vi "Enqueue--complete_tour_found.vi"(8 "error in (no error)":errorcluster, 11 "completed_tour":T1) -> (0 "error out":errorcluster)   [LabVIEW 2020, in "main.lvlib"]
doc: "Blank VI with error handling."
uses:
  main.lvlib
  core/core_data/completed_tour.ctl
  core/core_data/chessboard_index.ctl
  core/core_data/tour type (enum).ctl
  core/core_data/core_data.lvlib
panel:
  # "Development\ncontrols/indicators useful for development and testing, but which are not outputs of the VI"
  # "Input\nInputs to the VI"
  # "Output\nOutputs of the VI"
  # "Description\n\nBlank VI with error handling case. \n\nSummarize the use of this VI in this space."
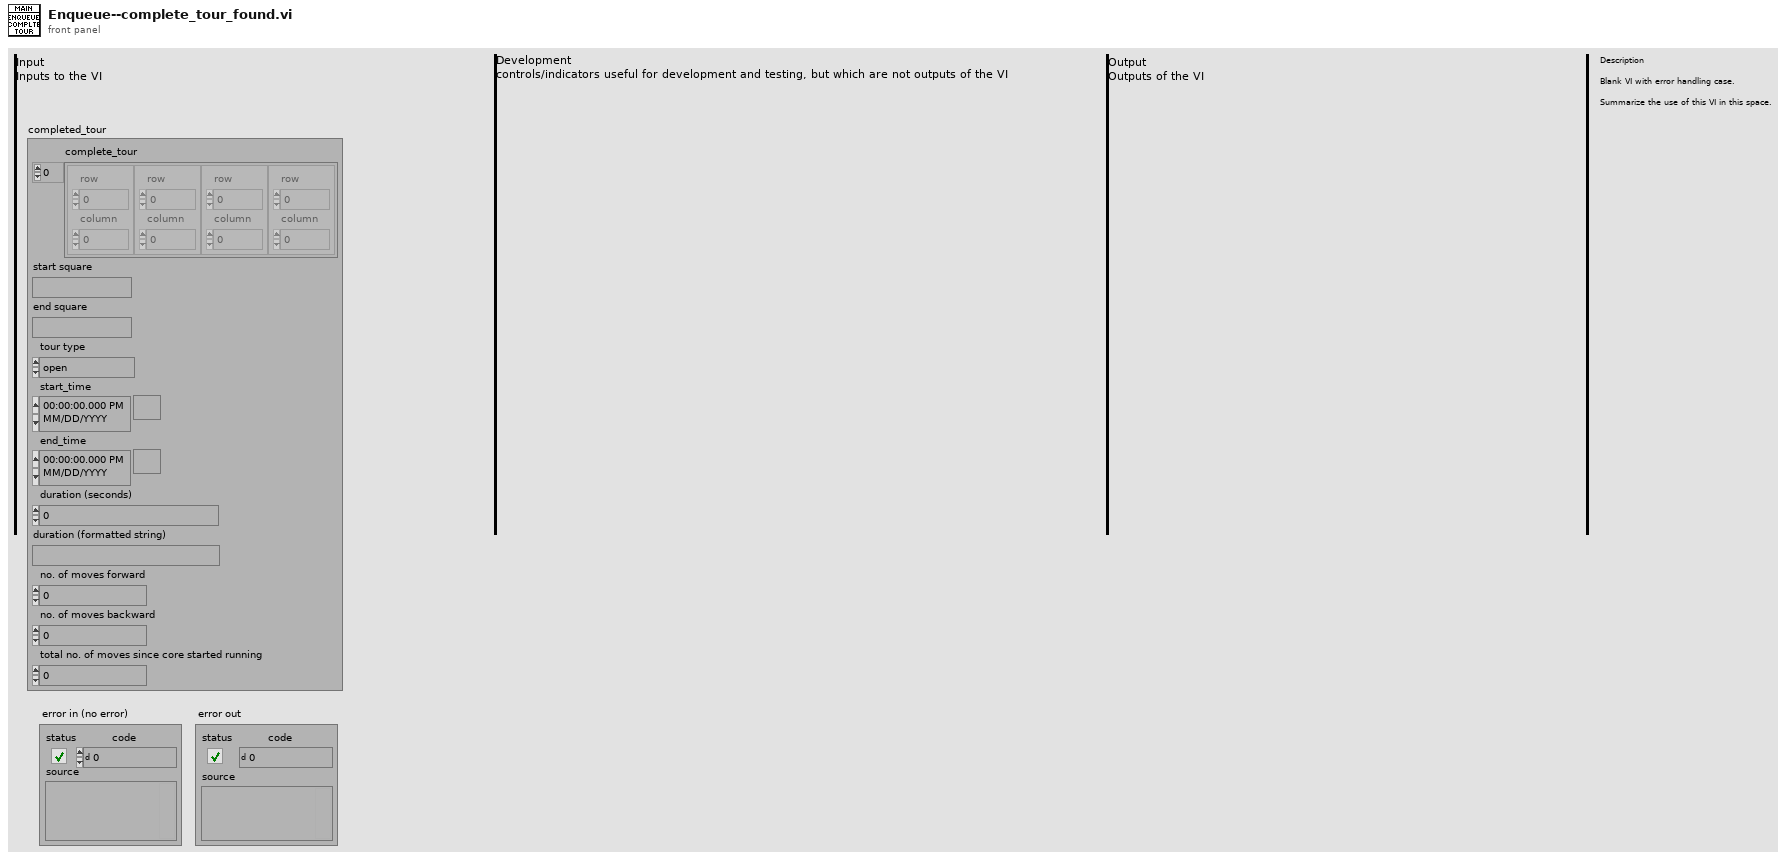
[diagram p1: front panel]
types:
  T1 = typedef "core.lvlib/core_data.lvlib/completed_tour.ctl" = cluster{"complete_tour":T2[], "start square":string, "end square":string, "tour type":T3, "start_time":timestamp, "end_time":timestamp, "duration (seconds)":dbl, "duration (formatted string)":string, "no. of moves forward":u64, "no. of moves backward":u64, "total no. of moves since core started running":u64}
  T2 = typedef "core.lvlib/core_data.lvlib/chessboard_index.ctl" = cluster{"row":u8, "column":u8}
  T3 = typedef "core.lvlib/core_data.lvlib/tour type (enum).ctl" = enum16{"open", "closed"}
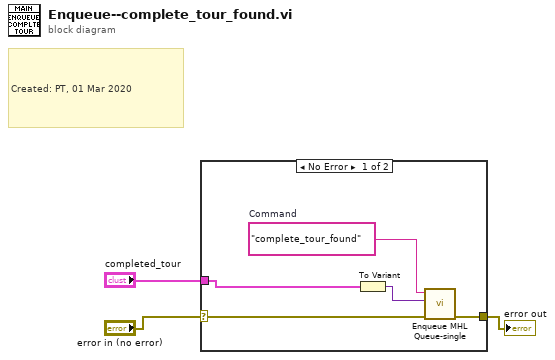
[diagram p0: block diagram]
diagram:
  # "Created: PT, 01 Mar 2020"
  n1 = case shown="No Error" "error in (no error)" {
    selector: "error in (no error)" -> [w7 w9]
    tunnel: [w6 w9] -> w2
    tunnel: "completed_tour" -> [w4 _]
    frame No Error {
      w8 = "complete_tour_found"  # Command
      n2 = To Variant(anything=w4) -> (Variant=w5:variant)
      n3 = call "Enqueue MHL Queue-single.vi"("ErrorIn"=w7, "Data"=w5, "Command"=w8) -> ("ErrorOut"=w6:errorcluster)  [unwired: 8 in]
    }
    frame Error {
    }
  }
  "error out" <- w2
